vi "Demo 1 - Image Gallery - Get Image Paths From Folder.vi"(8 "Error In":errorcluster, 11 "Image Folder Path In":path) -> (0 "Error Out":errorcluster, 3 "Image Paths Out":path[](array[path]))   [LabVIEW 2011]
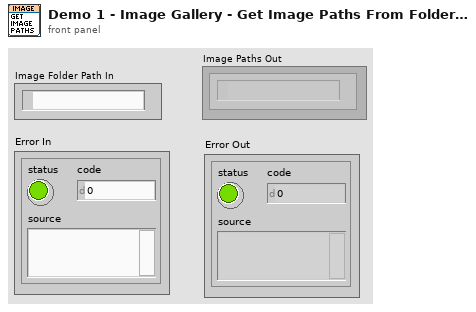
[diagram p1: front panel]
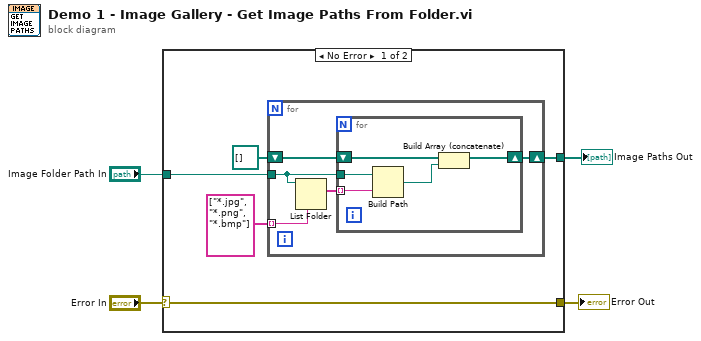
[diagram p0: block diagram]
diagram:
  n1 = case shown="No Error" "Error In" {
    selector: "Error In" -> [w5 w20]
    tunnel: "Image Folder Path In" -> [w9 _]
    tunnel: [w7 _] -> w3
    tunnel: [w5 w20] -> w1
    frame No Error {
      n2 = for {
        tunnel: w9 -> [w13]
        tunnel: string[] ["*.jpg", "*.png", "*.bmp"] -> [w14] mode=indexing
        shift-right: [w11] -> w7
        shift-left: path[] [] -> [w12]
        n3 = List Folder(path=w13, pattern=w14) -> (filenames=w10:string[])  [unwired: 2 in, 3 out]
        n4 = for {
          tunnel: w13 -> [w19]
          shift-right: [w16] -> w11
          shift-left: w12 -> [w17]
          tunnel: w10 -> [w15] mode=indexing
          n5 = Build Path(base path=w19, name or relative path=w15) -> (appended path=w18:path)
          n6 = Build Array (concatenate)(w17, w18) -> (w16:path[])
        }
      }
    }
    frame Error {
    }
  }
  "Image Paths Out" <- w3
  "Error Out" <- w1
